vi "Library Show Help.vi"() -> ()   [LabVIEW 2012]
doc: "This VI toggles the help window and its own window in which the description of the calling VI is displayed."
panel:
  out "description":string
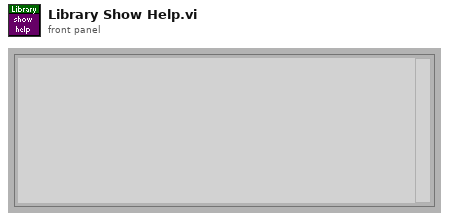
[diagram p1: front panel]
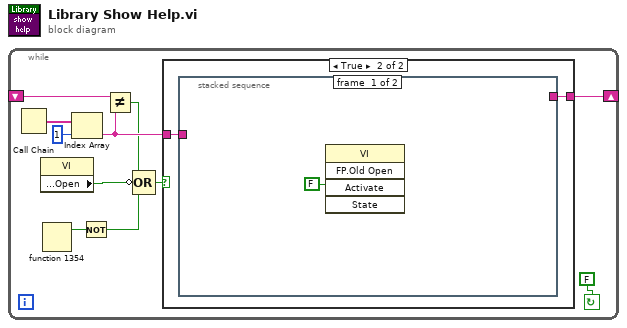
[diagram p0: block diagram]
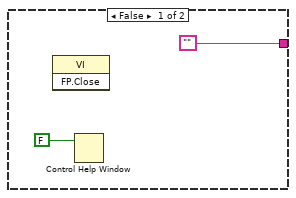
[diagram p2: hidden frame]
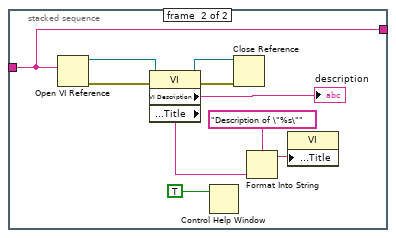
[diagram p3: hidden frame]
diagram:
  n1 = while {
    shift-left: _ -> [w9]
    shift-right: [w7] -> _
    stop <- FALSE continue-if-true
    n2 = Call Chain() -> (call chain=w11:string[])
    n3 = property class="VI"() -> ("Front Panel Window:Open"=w1:bool)  [unwired: 2 in, 2 out]
    n4 = fn#1354() -> (1:w4:bool)  [unwired: 1 out]
    n5 = Index Array(array=w11, index=1) -> (element=w8:string)
    n6 = Not(x=w4) -> (.not. x?=w3:bool)
    n7 = Not Equal?(x=w9, y=w8) -> (x != y?=w6:bool)
    n8 = Compound Arithmetic op=OR(w6, invert w1, w3) -> (w5:bool)
    n9 = case shown="True" w5 {
      tunnel: w8 -> [_ w15]
      tunnel: ["" w14] -> w7
      frame False {
        n10 = invoke class="VI" method="FP.Close"() -> ()  [unwired: 3 in, 3 out]
        n11 = Control Help Window(1:FALSE ("Show")) -> ()  [unwired: 1 in]
      }
      frame True {
        n12 = stacked-sequence {
          tunnel: w15 -> [_ w20]
          tunnel: [_ w20] -> w14
          frame #0 {
            n13 = invoke class="VI" method="FP.Old Open"("Activate"=FALSE) -> ()  [unwired: 4 in, 5 out]
          }
          frame #1 {
            n14 = Open VI Reference(vi path=w20) -> (vi reference=w25:refnum<vi>, error out=w26:errorcluster)  [unwired: 5 in]
            n15 = property class="VI"(reference=w25, error in=w26) -> (reference out=w18:refnum<vi>, error out=w19:errorcluster, "VI Description"=→"description":string, "Front Panel Window:Title"=w21:string)
            n16 = Control Help Window(1:TRUE ("Show")) -> ()  [unwired: 1 in]
            n17 = Close Reference(reference=w18, error in (no error)=w19) -> ()  [unwired: 1 out]
            n18 = Format Into String(format string="Description of \"%s\"" ("Format String"), w21) -> (resulting string=w17:string)  [unwired: 2 in, 1 out]
            n19 = property class="VI"("Front Panel Window:Title"=w17) -> ()  [unwired: 2 in, 2 out]
          }
        }
      }
    }
  }
